vi "add_vehicle_settings.vi"(4 "vehicle_settings":T1={"enable"=0, "run"=0, "gui_connection_required"=1, "max_speed"=3.0}, 5 "msg in":string) -> (2 "msg out":string)   [LabVIEW 2016]
uses:
  <userlib>/ROS for LabVIEW Software/ROS/MessageBuilding/std_msgs/subs/i8Scalar.vi
  <userlib>/ROS for LabVIEW Software/ROS/MessageBuilding/std_msgs/subs/float64Scalar.vi
  <userlib>/ROS for LabVIEW Software/ROS/MessageBuilding/std_msgs/subs/timeScalar.vi
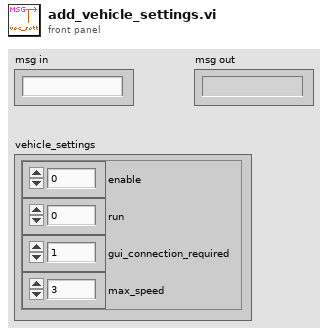
[diagram p1: front panel]
types:
  T1 = cluster{"enable":i8, "run":i8, "gui_connection_required":i8, "max_speed":dbl}
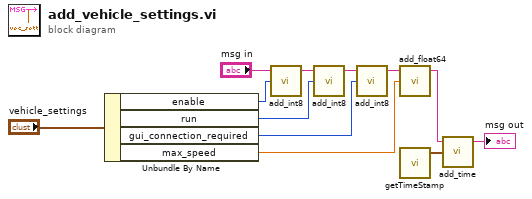
[diagram p0: block diagram]
diagram:
  n1 = Unbundle By Name("vehicle_settings") -> ("enable"=w6:i8, "run"=w5:i8, "gui_connection_required"=w4:i8, "max_speed"=w2:dbl)
  n2 = call-poly <userlib>:"add_int8.vi"("Numeric"=w6, "msg in"="msg in") -> ("msg out"=w11:string)  [unwired: 3 in]
  n3 = call-poly <userlib>:"add_int8.vi"("Numeric"=w5, "msg in"=w11) -> ("msg out"=w3:string)  [unwired: 3 in]
  n4 = call-poly <userlib>:"add_int8.vi"("Numeric"=w4, "msg in"=w3) -> ("msg out"=w10:string)  [unwired: 3 in]
  n5 = call-poly <userlib>:"add_float64.vi"("Numeric"=w2, "msg in"=w10) -> ("msg out"=w9:string)  [unwired: 3 in]
  n6 = call <userlib>:"getTimeStamp.vi"() -> ("ROS Time"=w1:cluster{"secs":i32, "nsecs":i32})  [unwired: 2 in, 2 out]
  n7 = call-poly <userlib>:"add_time.vi"("Time"=w1, "msg in"=w9) -> ("msg out"=→"msg out":string)  [unwired: 3 in]
